vi "Pytagore.vi"   [LabVIEW 2011]
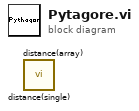
[diagram p0: block diagram]
diagram:
  n1 = call "distance(single).vi"() -> ()  [unwired: 2 in, 1 out]
  n2 = call "distance(array).vi"() -> ()  [unwired: 2 in, 1 out]
